vi "FTW-TestExecutive-Core_Step_Launch.vi"(0 "FTW-TestExecutive-Core In":refnum<class "FTW-TestExecutive-Core.lvclass">, 11 "error in":errorcluster) -> (4 "FTW-TestExecutive-Core Out":refnum<class "FTW-TestExecutive-Core.lvclass">, 15 "error out":errorcluster)   [LabVIEW 2015, in "FTW-TestExecutive-Core.lvclass"]
uses:
  FTW-TestExecutive-Core.lvclass
  source/actor/Connector/FTW-ActorConnector.lvclass
  FTW-TestExecutive-Core.lvclass/FTW-TestExecutive-Core.ctl
  source/actor/Instance/FTW-ActorInstance.lvclass/FTW-ActorInstance.ctl
  source/JSON/core/FTW-JSON-Core-EncodingFlags.vi
  source/JSON/FTW-JSON-Parse.vi
  source/Reflection/FTW-Reflection-Type.vi
  source/CodeGen/JSON Deserialize/FTW-JSON-Core-GetFlattenedValue.vi
  source/CodeGen/JSON Deserialize/FTW-JSON-Deserialize.xnode
  source/actor/Instance/FTW-ActorInstance.lvclass
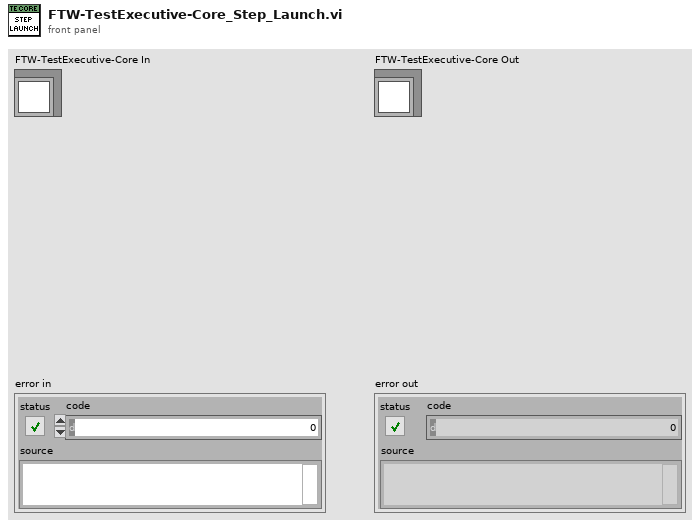
[diagram p1: front panel]
types:
  T1 = typedef "FTW-TestExecutive-Step.ctl" = cluster{"Name":string, "Type":string, "Config":string, "Elapsed Time":dbl, "Passed":bool, "State":T2, "Results":T3}
  T2 = typedef "FTW-TestExecutive-Step-State.ctl" = enum8{"None", "Failed", "Passed", "Timed out", "Aborted"}
  T3 = typedef "FTW-TestExecutive-Results.ctl" = cluster{"Start Time":timestamp, "Elapsed Time":dbl, "Passed":bool}
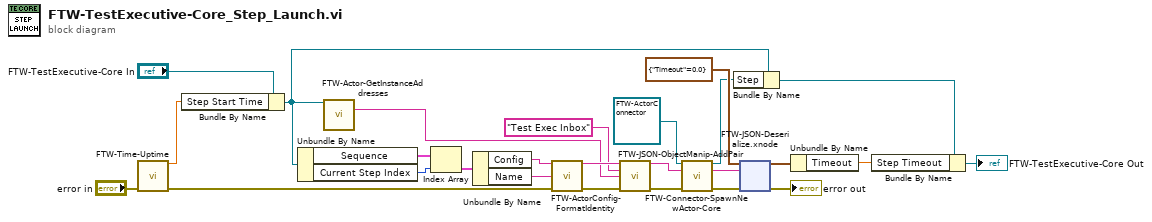
[diagram p0: block diagram]
diagram:
  n1 = call "FTW-Time-Uptime.vi"("error in"="error in") -> ("Current Uptime"=w20:dbl, "error out"=w21:errorcluster)  [unwired: 12 in, 1 out]
  n2 = Bundle By Name(cluster="FTW-TestExecutive-Core In", "Step Start Time"=w20) -> (w5:refnum<class "FTW-TestExecutive-Core.lvclass">)
  n3 = Unbundle By Name(w5) -> ("Sequence"=w26:T1[], "Current Step Index"=w25:i32)
  n4 = call "FTW-Actor-GetInstanceAddresses.vi"("FTW Actor Instance"=w5) -> ("Inbox Address"=w7:string)  [unwired: 12 in, 2 out]
  n5 = Index Array(array=w26, index=w25) -> (element=w24:T1)
  n6 = Unbundle By Name(w24) -> ("Config"=w13:string, "Name"=w12:string)
  n7 = call "FTW-ActorConfig-FormatIdentity.vi"("FTW Config String In"=w13, "Identity"=w12, "error in"=w21) -> ("FTW Config String"=w10:string, "error out"=w14:errorcluster)  [unwired: 11 in]
  n8 = call "FTW-JSON-ObjectManip-AddPair.vi"("Input JSON Object"=w10, "Key"="Test Exec Inbox", "Value"=w7, "error in"=w14) -> ("Output JSON Object"=w9:string, "error out"=w11:errorcluster)  [unwired: 10 in]
  n9 = call "FTW-Connector-SpawnNewActor-Core.vi"("FTW Actor Connector Type"=refnum<class "FTW-ActorConnector.lvclass"> refnum, "Configuration"=w9, "error in"=w11) -> ("FTW Actor Connector"=w2:refnum<class "FTW-ActorConnector.lvclass">, "Initialized Response"=w1:string, "error out"=w6:errorcluster)  [unwired: 9 in, 1 out]
  n10 = Bundle By Name(cluster=w5, "Step"=w2) -> (w4:refnum<class "FTW-TestExecutive-Core.lvclass">)
  n11 = xnode "FTW-JSON-Deserialize.xnode"("Type and Defaults"=cluster{"Timeout":dbl} {"Timeout"=0.0}, "JSON String"=w1, "error in"=w6) -> ("Values"=w16:cluster{"Timeout":dbl}, "error out"=→"error out":errorcluster)
  n12 = Unbundle By Name(w16) -> ("Timeout"=w15:dbl)
  n13 = Bundle By Name(cluster=w4, "Step Timeout"=w15) -> (→"FTW-TestExecutive-Core Out":refnum<class "FTW-TestExecutive-Core.lvclass">)
